vi "Read Config File Path.vi"(11 "Process In":refnum<class "Process.lvclass">) -> (2 "Config File Path":path, 3 "Process Out":refnum<class "Process.lvclass">)   [LabVIEW 2020, in "Process.lvclass"]
uses:
  Process.lvclass
  Process.lvclass/Process.ctl
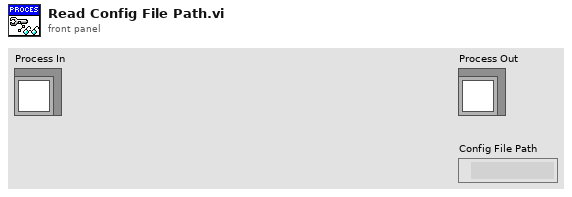
[diagram p1: front panel]
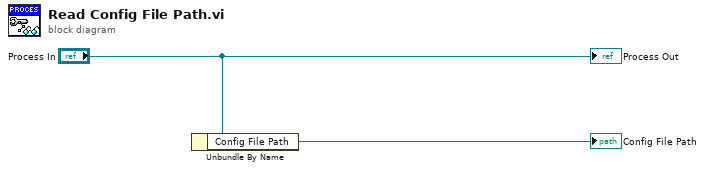
[diagram p0: block diagram]
diagram:
  n1 = Unbundle By Name("Process In") -> ("Config File Path"=→"Config File Path":path)
  "Process Out" <- "Process In"
